vi "Radians to Direction.vi"(11 "Radian Heading (0 = East)":dbl) -> (3 "Closest Direction":T1)   [LabVIEW 2020, in "SquareBattle.lvlib"]
doc: "Returns the closest direction enumeration to the specified direction in radians. Note that 0 radians is equivalent to due East similar to if ATAN was used to return the heading from x and y components."
uses:
  SquareBattle.lvlib
  Direction.ctl
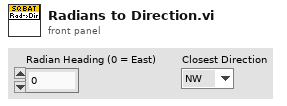
[diagram p1: front panel]
types:
  T1 = typedef "SquareBattle.lvlib/Direction.ctl" = enum16{"NW", "N", "NE", "E", "SE", "S", "SW", "W"}
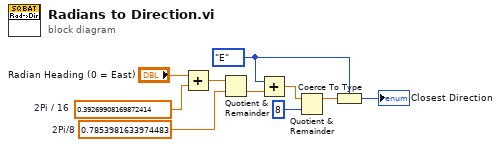
[diagram p0: block diagram]
diagram:
  w1 = Direction."E" ("Direction")
  w7 = 0.7853981633974483  # 2Pi/8
  w9 = 0.39269908169872414  # 2Pi / 16
  n1 = Add(x="Radian Heading (0 = East)", y=w9) -> (x+y=w8:dbl)
  n2 = Quotient & Remainder(x=w8, y=w7) -> (floor(x/y)=w6:dbl)  [unwired: 1 out]
  n3 = Add(x=w1, y=w6) -> (x+y=w5:dbl)
  n4 = Quotient & Remainder(x=w5, y=8 ("32bit integer")) -> (x-y*floor(x/y)=w3:dbl)  [unwired: 1 out]
  n5 = Coerce To Type(0:w3, 1:w1) -> (2:→"Closest Direction":T1)
